vi "Decode.vi"(8 "Inputs":T1={"Frequency1"=2000.0, "Bit Duration in ms"=0.05, "Frequency2"=4000.0, "Amplitude Scale"=1.0, "Sampling Rate"=50000} {"Frequency2" format="%#_13g"; "Frequency1" format="%#_13g"}, 10 "Waveform Array":u16[](array[numeric])=array[20000 elements], 11 "Expected Characters":u16) -> (2 "string":string)   [LabVIEW 2021]
uses:
  <vilib>/Analysis/baseanly.llb/Mean (DBL).vi
  <vilib>/Analysis/NI_AALBase.lvlib
panel:
  out "size(s)":i32
  out "Array":bool[](array[boolean])
  out "Samples per bit":dbl
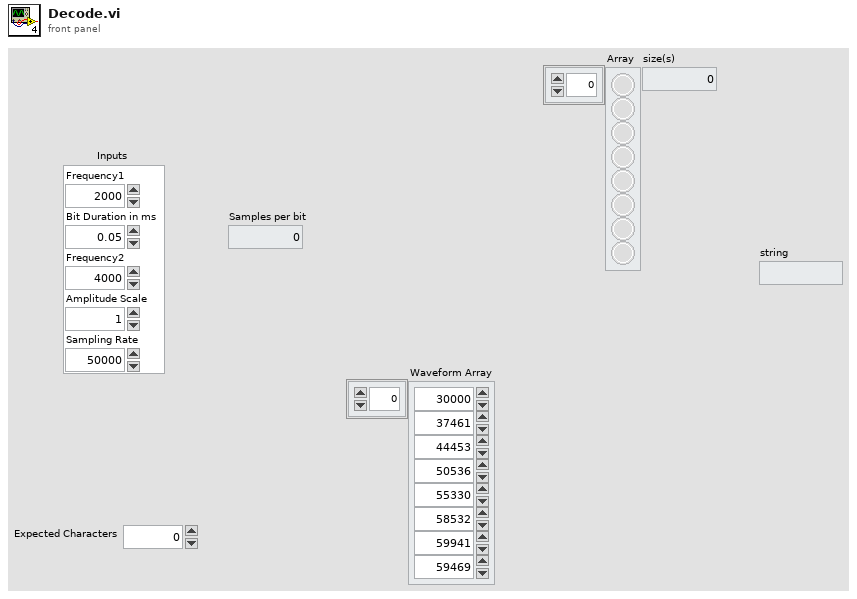
[diagram p1: front panel]
types:
  T1 = cluster{"Frequency1":dbl, "Bit Duration in ms":dbl, "Frequency2":dbl, "Amplitude Scale":dbl, "Sampling Rate":u32}
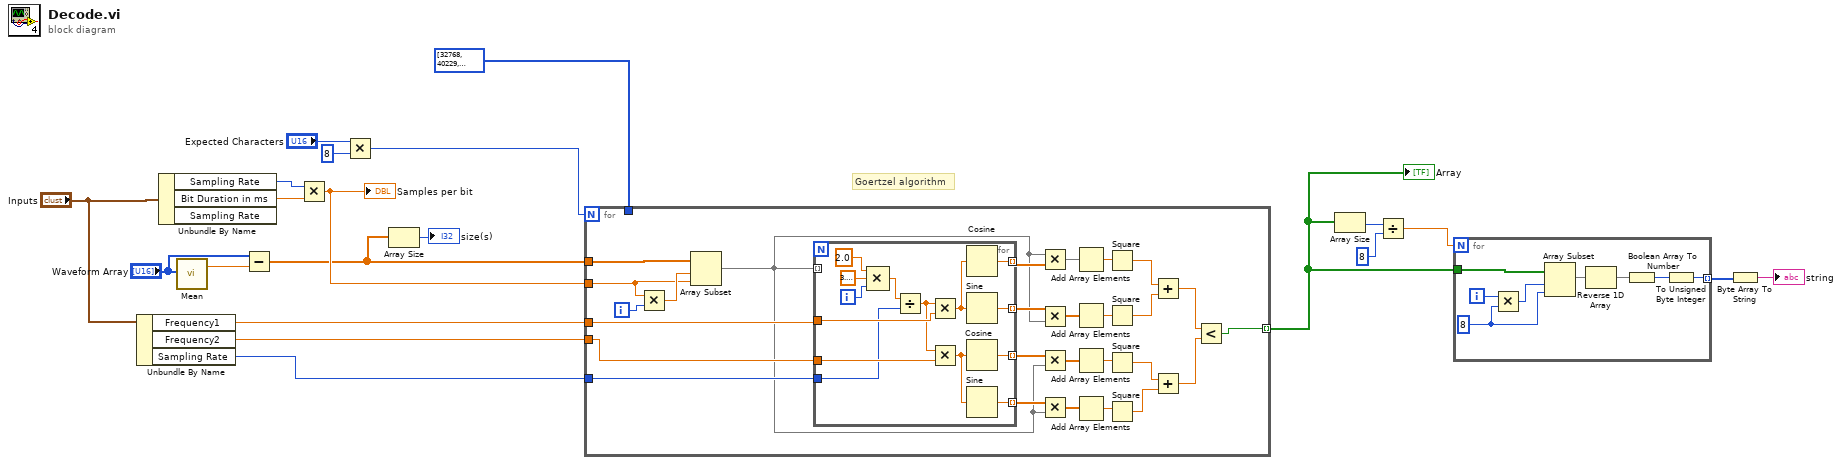
[diagram p0: block diagram]
diagram:
  # "Goertzel algorithm"
  n1 = Unbundle By Name("Inputs") -> ("Frequency1"=w15:dbl, "Frequency2"=w14:dbl, "Sampling Rate"=w13:u32)
  n2 = Unbundle By Name("Inputs") -> ("Sampling Rate"=w19:u32, "Bit Duration in ms"=w18:dbl)  [unwired: 1 out]
  n3 = call-poly <vilib>:"Mean.vi"("X"="Waveform Array") -> ("mean"=w20:dbl)  [unwired: 1 out]
  n4 = Subtract(x="Waveform Array", y=w20) -> (x-y=w6:dbl[])
  n5 = Multiply(x=w19, y=w18) -> (x*y=w17:dbl)
  "Samples per bit" <- w17
  n6 = Multiply(x="Expected Characters", y=u16 8) -> (x*y=w2:u16)
  n7 = Array Size(array=w6) -> (size(s)=→"size(s)":i32)
  n8 = for {
    N: w2 -> [_]
    tunnel: w6 -> [w48]
    tunnel: w17 -> [w45]
    tunnel: w15 -> [w43]
    tunnel: w14 -> [w44]
    tunnel: w13 -> [w42]
    tunnel: [w22] -> w12 mode=indexing
    tunnel: u16[] [32768, 40229, 47221, 53304, 58098, 61300, 62709, 62237, 59913, 55883, 50402, 43812, 36528, 29008, 21724, 15134, 9653, 5623, 3299, 2827, 4236, 7438, 12232, 18315, 25307, 32768, 40229, 47221, 53304, 58098, 61300, 62709, 62237, 59913, 55883, 50402, 43812, 36528, 29008, 21724, 15134, 9653, 5623, 3299, 2827, 4236, 7438, 12232, 18315, 25307, 32768, 40229, 47221, 53304, 58098, 61300, 62709, 62237, 59913, 55883, 50402, 43812, 36528, 29008, 21724, 15134, 9653, 5623, 3299, 2827, 4236, 7438, 12232, 18315, 25307, 32768, 40229, 47221, 53304, 58098, 61300, 62709, 62237, 59913, 55883, 50402, 43812, 36528, 29008, 21724, 15134, 9653, 5623, 3299, 2827, 4236, 7438, 12232, 18315, 25307, 32768, 40229, 47221, 53304, 58098, 61300, 62709, 62237, 59913, 55883, 50402, 43812, 36528, 29008, 21724, 15134, 9653, 5623, 3299, 2827, 4236, 7438, 12232, 18315, 25307, 32768, 40229, 47221, 53304, 58098, 61300, 62709, 62237, 59913, 55883, 50402, 43812, 36528, 29008, 21724, 15134, 9653, 5623, 3299, 2827, 4236, 7438, 12232, 18315, 25307, 32768, 40229, 47221, 53304, 58098, 61300, 62709, 62237, 59913, 55883, 50402, 43812, 36528, 29008, 21724, 15134, 9653, 5623, 3299, 2827, 4236, 7438, 12232, 18315, 25307, 32768, 40229, 47221, 53304, 58098, 61300, 62709, 62237, 59913, 55883, 50402, 43812, 36528, 29008, 21724, 15134, 9653, 5623, 3299, 2827, 4236, 7438, 12232, 18315, 25307, 32768, 40229, 47221, 53304, 58098, 61300, 62709, 62237, 59913, 55883, 50402, 43812, 36528, 29008, 21724, 15134, 9653, 5623, 3299, 2827, 4236, 7438, 12232, 18315, 25307, 32768, 40229, 47221, 53304, 58098, 61300, 62709, 62237, 59913, 55883, 50402, 43812, 36528, 29008, 21724, 15134, 9653, 5623, 3299, 2827, 4236, 7438, 12232, 18315, 25307, 32768, 40229, 47221, 53304, 58098, 61300, 62709, 62237, 59913, 55883, 50402, 43812, 36528, 29008, 21724, 15134, 9653, 5623, 3299, 2827, 4236, 7438, 12232, 18315, 25307, 32768, 40229, 47221, 53304, 58098, 61300, 62709, 62237, 59913, 55883, 50402, 43812, 36528, 29008, 21724, 15134, 9653, 5623, 3299, 2827, 4236, 7438, 12232, 18315, 25307, 32768, 40229, 47221, 53304, 58098, 61300, 62709, 62237, 59913, 55883, 50402, 43812, 36528, 29008, 21724, 15134, 9653, 5623, 3299, 2827, 4236, 7438, 12232, 18315, 25307, 32768, 40229, 47221, 53304, 58098, 61300, 62709, 62237, 59913, 55883, 50402, 43812, 36528, 29008, 21724, 15134, 9653, 5623, 3299, 2827, 4236, 7438, 12232, 18315, 25307, 32768, 40229, 47221, 53304, 58098, 61300, 62709, 62237, 59913, 55883, 50402, 43812, 36528, 29008, 21724, 15134, 9653, 5623, 3299, 2827, 4236, 7438, 12232, 18315, 25307, 32768, 40229, 47221, 53304, 58098, 61300, 62709, 62237, 59913, 55883, 50402, 43812, 36528, 29008, 21724, 15134, 9653, 5623, 3299, 2827, 4236, 7438, 12232, 18315, 25307, 32768, 40229, 47221, 53304, 58098, 61300, 62709, 62237, 59913, 55883, 50402, 43812, 36528, 29008, 21724, 15134, 9653, 5623, 3299, 2827, 4236, 7438, 12232, 18315, 25307, 32768, 40229, 47221, 53304, 58098, 61300, 62709, 62237, 59913, 55883, 50402, 43812, 36528, 29008, 21724, 15134, 9653, 5623, 3299, 2827, 4236, 7438, 12232, 18315, 25307, 32768, 40229, 47221, 53304, 58098, 61300, 62709, 62237, 59913, 55883, 50402, 43812, 36528, 29008, 21724, 15134, 9653, 5623, 3299, 2827, 4236, 7438, 12232, 18315, 25307, 32768, 40229, 47221, 53304, 58098, 61300, 62709, 62237, 59913, 55883, 50402, 43812, 36528, 29008, 21724, 15134, 9653, 5623, 3299, 2827, 4236, 7438, 12232, 18315, 25307, 32768, 40229, 47221, 53304, 58098, 61300, 62709, 62237, 59913, 55883, 50402, 43812, 36528, 29008, 21724, 15134, 9653, 5623, 3299, 2827, 4236, 7438, 12232, 18315, 25307, 32768, 40229, 47221, 53304, 58098, 61300, 62709, 62237, 59913, 55883, 50402, 43812, 36528, 29008, 21724, 15134, 9653, 5623, 3299, 2827, 4236, 7438, 12232, 18315, 25307, 32768, 40229, 47221, 53304, 58098, 61300, 62709, 62237, 59913, 55883, 50402, 43812, 36528, 29008, 21724, 15134, 9653, 5623, 3299, 2827, 4236, 7438, 12232, 18315, 25307, 32768, 40229, 47221, 53304, 58098, 61300, 62709, 62237, 59913, 55883, 50402, 43812, 36528, 29008, 21724, 15134, 9653, 5623, 3299, 2827, 4236, 7438, 12232, 18315, 25307, 32768, 40229, 47221, 53304, 58098, 61300, 62709, 62237, 59913, 55883, 50402, 43812, 36528, 29008, 21724, 15134, 9653, 5623, 3299, 2827, 4236, 7438, 12232, 18315, 25307, 32768, 40229, 47221, 53304, 58098, 61300, 62709, 62237, 59913, 55883, 50402, 43812, 36528, 29008, 21724, 15134, 9653, 5623, 3299, 2827, 4236, 7438, 12232, 18315, 25307, 32768, 40229, 47221, 53304, 58098, 61300, 62709, 62237, 59913, 55883, 50402, 43812, 36528, 29008, 21724, 15134, 9653, 5623, 3299, 2827, 4236, 7438, 12232, 18315, 25307, 32768, 40229, 47221, 53304, 58098, 61300, 62709, 62237, 59913, 55883, 50402, 43812, 36528, 29008, 21724, 15134, 9653, 5623, 3299, 2827, 4236, 7438, 12232, 18315, 25307, 32768, 40229, 47221, 53304, 58098, 61300, 62709, 62237, 59913, 55883, 50402, 43812, 36528, 29008, 21724, 15134, 9653, 5623, 3299, 2827, 4236, 7438, 12232, 18315, 25307, 32768, 40229, 47221, 53304, 58098, 61300, 62709, 62237, 59913, 55883, 50402, 43812, 36528, 29008, 21724, 15134, 9653, 5623, 3299, 2827, 4236, 7438, 12232, 18315, 25307, 32768, 40229, 47221, 53304, 58098, 61300, 62709, 62237, 59913, 55883, 50402, 43812, 36528, 29008, 21724, 15134, 9653, 5623, 3299, 2827, 4236, 7438, 12232, 18315, 25307, 32768, 40229, 47221, 53304, 58098, 61300, 62709, 62237, 59913, 55883, 50402, 43812, 36528, 29008, 21724, 15134, 9653, 5623, 3299, 2827, 4236, 7438, 12232, 18315, 25307, 32768, 40229, 47221, 53304, 58098, 61300, 62709, 62237, 59913, 55883, 50402, 43812, 36528, 29008, 21724, 15134, 9653, 5623, 3299, 2827, 4236, 7438, 12232, 18315, 25307, 32768, 40229, 47221, 53304, 58098, 61300, 62709, 62237, 59913, 55883, 50402, 43812, 36528, 29008, 21724, 15134, 9653, 5623, 3299, 2827, 4236, 7438, 12232, 18315, 25307, 32768, 40229, 47221, 53304, 58098, 61300, 62709, 62237, 59913, 55883, 50402, 43812, 36528, 29008, 21724, 15134, 9653, 5623, 3299, 2827, 4236, 7438, 12232, 18315, 25307, 32768, 40229, 47221, 53304, 58098, 61300, 62709, 62237, 59913, 55883, 50402, 43812, 36528, 29008, 21724, 15134, 9653, 5623, 3299, 2827, 4236, 7438, 12232, 18315, 25307, 32768, 40229, 47221, 53304, 58098, 61300, 62709, 62237, 59913, 55883, 50402, 43812, 36528, 29008, 21724, 15134, 9653, 5623, 3299, 2827, 4236, 7438, 12232, 18315, 25307, 32768, 40229, 47221, 53304, 58098, 61300, 62709, 62237, 59913, 55883, 50402, 43812, 36528, 29008, 21724, 15134, 9653, 5623, 3299, 2827, 4236, 7438, 12232, 18315, 25307, 32768, 40229, 47221, 53304, 58098, 61300, 62709, 62237, 59913, 55883, 50402, 43812, 36528, 29008, 21724, 15134, 9653, 5623, 3299, 2827, 4236, 7438, 12232, 18315, 25307, 32768, 40229, 47221, 53304, 58098, 61300, 62709, 62237, 59913, 55883, 50402, 43812, 36528, 29008, 21724, 15134, 9653, 5623, 3299, 2827, 4236, 7438, 12232, 18315, 25307, 32768, 40229, 47221, 53304, 58098, 61300, 62709, 62237, 59913, 55883, 50402, 43812, 36528, 29008, 21724, 15134, 9653, 5623, 3299, 2827, 4236, 7438, 12232, 18315, 25307, 32768, 40229, 47221, 53304, 58098, 61300, 62709, 62237, 59913, 55883, 50402, 43812, 36528, 29008, 21724, 15134, 9653, 5623, 3299, 2827, 4236, 7438, 12232, 18315, 25307, 32768, 40229, 47221, 53304, 58098, 61300, 62709, 62237, 59913, 55883, 50402, 43812, 36528, 29008, 21724, 15134, 9653, 5623, 3299, 2827, 4236, 7438, 12232, 18315, 25307, 32768, 40229, 47221, 53304, 58098, 61300, 62709, 62237, 59913, 55883, 50402, 43812, 36528, 29008, 21724, 15134, 9653, 5623, 3299, 2827, 4236, 7438, 12232, 18315, 25307, 32768, 40229, 47221, 53304, 58098, 61300, 62709, 62237, 59913, 55883, 50402, 43812, 36528, 29008, 21724, 15134, 9653, 5623, 3299, 2827, 4236, 7438, 12232, 18315, 25307, 32768, 40229, 47221, 53304, 58098, 61300, 62709, 62237, 59913, 55883, 50402, 43812, 36528, 29008, 21724, 15134, 9653, 5623, 3299, 2827, 4236, 7438, 12232, 18315, 25307, 32768, 40229, 47221, 53304, 58098, 61300, 62709, 62237, 59913, 55883, 50402, 43812, 36528, 29008, 21724, 15134, 9653, 5623, 3299, 2827, 4236, 7438, 12232, 18315, 25307, 32768, 40229, 47221, 53304, 58098, 61300, 62709, 62237, 59913, 55883, 50402, 43812, 36528, 29008, 21724, 15134, 9653, 5623, 3299, 2827, 4236, 7438, 12232, 18315, 25307, 32768, 40229, 47221, 53304, 58098, 61300, 62709, 62237, 59913, 55883, 50402, 43812, 36528, 29008, 21724, 15134, 9653, 5623, 3299, 2827, 4236, 7438, 12232, 18315, 25307, 32768, 40229, 47221, 53304, 58098, 61300, 62709, 62237, 59913, 55883, 50402, 43812, 36528, 29008, 21724, 15134, 9653, 5623, 3299, 2827, 4236, 7438, 12232, 18315, 25307, 32768, 40229, 47221, 53304, 58098, 61300, 62709, 62237, 59913, 55883, 50402, 43812, 36528, 29008, 21724, 15134, 9653, 5623, 3299, 2827, 4236, 7438, 12232, 18315, 25307, 32768, 40229, 47221, 53304, 58098, 61300, 62709, 62237, 59913, 55883, 50402, 43812, 36528, 29008, 21724, 15134, 9653, 5623, 3299, 2827, 4236, 7438, 12232, 18315, 25307, 32768, 40229, 47221, 53304, 58098, 61300, 62709, 62237, 59913, 55883, 50402, 43812, 36528, 29008, 21724, 15134, 9653, 5623, 3299, 2827, 4236, 7438, 12232, 18315, 25307, 32768, 40229, 47221, 53304, 58098, 61300, 62709, 62237, 59913, 55883, 50402, 43812, 36528, 29008, 21724, 15134, 9653, 5623, 3299, 2827, 4236, 7438, 12232, 18315, 25307, 32768, 40229, 47221, 53304, 58098, 61300, 62709, 62237, 59913, 55883, 50402, 43812, 36528, 29008, 21724, 15134, 9653, 5623, 3299, 2827, 4236, 7438, 12232, 18315, 25307, 32768, 40229, 47221, 53304, 58098, 61300, 62709, 62237, 59913, 55883, 50402, 43812, 36528, 29008, 21724, 15134, 9653, 5623, 3299, 2827, 4236, 7438, 12232, 18315, 25307, 32768, 40229, 47221, 53304, 58098, 61300, 62709, 62237, 59913, 55883, 50402, 43812, 36528, 29008, 21724, 15134, 9653, 5623, 3299, 2827, 4236, 7438, 12232, 18315, 25307, 32768, 40229, 47221, 53304, 58098, 61300, 62709, 62237, 59913, 55883, 50402, 43812, 36528, 29008, 21724, 15134, 9653, 5623, 3299, 2827, 4236, 7438, 12232, 18315, 25307, 32768, 40229, 47221, 53304, 58098, 61300, 62709, 62237, 59913, 55883, 50402, 43812, 36528, 29008, 21724, 15134, 9653, 5623, 3299, 2827, 4236, 7438, 12232, 18315, 25307, 32768, 40229, 47221, 53304, 58098, 61300, 62709, 62237, 59913, 55883, 50402, 43812, 36528, 29008, 21724, 15134, 9653, 5623, 3299, 2827, 4236, 7438, 12232, 18315, 25307, 32768, 40229, 47221, 53304, 58098, 61300, 62709, 62237, 59913, 55883, 50402, 43812, 36528, 29008, 21724, 15134, 9653, 5623, 3299, 2827, 4236, 7438, 12232, 18315, 25307, 32768, 40229, 47221, 53304, 58098, 61300, 62709, 62237, 59913, 55883, 50402, 43812, 36528, 29008, 21724, 15134, 9653, 5623, 3299, 2827, 4236, 7438, 12232, 18315, 25307, 32768, 40229, 47221, 53304, 58098, 61300, 62709, 62237, 59913, 55883, 50402, 43812, 36528, 29008, 21724, 15134, 9653, 5623, 3299, 2827, 4236, 7438, 12232, 18315, 25307, 32768, 40229, 47221, 53304, 58098, 61300, 62709, 62237, 59913, 55883, 50402, 43812, 36528, 29008, 21724, 15134, 9653, 5623, 3299, 2827, 4236, 7438, 12232, 18315, 25307, 32768, 40229, 47221, 53304, 58098, 61300, 62709, 62237, 59913, 55883, 50402, 43812, 36528, 29008, 21724, 15134, 9653, 5623, 3299, 2827, 4236, 7438, 12232, 18315, 25307, 32768, 40229, 47221, 53304, 58098, 61300, 62709, 62237, 59913, 55883, 50402, 43812, 36528, 29008, 21724, 15134, 9653, 5623, 3299, 2827, 4236, 7438, 12232, 18315, 25307, 32768, 40229, 47221, 53304, 58098, 61300, 62709, 62237, 59913, 55883, 50402, 43812, 36528, 29008, 21724, 15134, 9653, 5623, 3299, 2827, 4236, 7438, 12232, 18315, 25307, 32768, 40229, 47221, 53304, 58098, 61300, 62709, 62237, 59913, 55883, 50402, 43812, 36528, 29008, 21724, 15134, 9653, 5623, 3299, 2827, 4236, 7438, 12232, 18315, 25307, 32768, 40229, 47221, 53304, 58098, 61300, 62709, 62237, 59913, 55883, 50402, 43812, 36528, 29008, 21724, 15134, 9653, 5623, 3299, 2827, 4236, 7438, 12232, 18315, 25307, 32768, 40229, 47221, 53304, 58098, 61300, 62709, 62237, 59913, 55883, 50402, 43812, 36528, 29008, 21724, 15134, 9653, 5623, 3299, 2827, 4236, 7438, 12232, 18315, 25307, 32768, 40229, 47221, 53304, 58098, 61300, 62709, 62237, 59913, 55883, 50402, 43812, 36528, 29008, 21724, 15134, 9653, 5623, 3299, 2827, 4236, 7438, 12232, 18315, 25307, 32768, 40229, 47221, 53304, 58098, 61300, 62709, 62237, 59913, 55883, 50402, 43812, 36528, 29008, 21724, 15134, 9653, 5623, 3299, 2827, 4236, 7438, 12232, 18315, 25307, 32768, 40229, 47221, 53304, 58098, 61300, 62709, 62237, 59913, 55883, 50402, 43812, 36528, 29008, 21724, 15134, 9653, 5623, 3299, 2827, 4236, 7438, 12232, 18315, 25307, 32768, 40229, 47221, 53304, 58098, 61300, 62709, 62237, 59913, 55883, 50402, 43812, 36528, 29008, 21724, 15134, 9653, 5623, 3299, 2827, 4236, 7438, 12232, 18315, 25307, 32768, 40229, 47221, 53304, 58098, 61300, 62709, 62237, 59913, 55883, 50402, 43812, 36528, 29008, 21724, 15134, 9653, 5623, 3299, 2827, 4236, 7438, 12232, 18315, 25307, 32768, 40229, 47221, 53304, 58098, 61300, 62709, 62237, 59913, 55883, 50402, 43812, 36528, 29008, 21724, 15134, 9653, 5623, 3299, 2827, 4236, 7438, 12232, 18315, 25307, 32768, 40229, 47221, 53304, 58098, 61300, 62709, 62237, 59913, 55883, 50402, 43812, 36528, 29008, 21724, 15134, 9653, 5623, 3299, 2827, 4236, 7438, 12232, 18315, 25307, 32768, 40229, 47221, 53304, 58098, 61300, 62709, 62237, 59913, 55883, 50402, 43812, 36528, 29008, 21724, 15134, 9653, 5623, 3299, 2827, 4236, 7438, 12232, 18315, 25307, 32768, 40229, 47221, 53304, 58098, 61300, 62709, 62237, 59913, 55883, 50402, 43812, 36528, 29008, 21724, 15134, 9653, 5623, 3299, 2827, 4236, 7438, 12232, 18315, 25307, 32768, 40229, 47221, 53304, 58098, 61300, 62709, 62237, 59913, 55883, 50402, 43812, 36528, 29008, 21724, 15134, 9653, 5623, 3299, 2827, 4236, 7438, 12232, 18315, 25307, 32768, 40229, 47221, 53304, 58098, 61300, 62709, 62237, 59913, 55883, 50402, 43812, 36528, 29008, 21724, 15134, 9653, 5623, 3299, 2827, 4236, 7438, 12232, 18315, 25307, 32768, 40229, 47221, 53304, 58098, 61300, 62709, 62237, 59913, 55883, 50402, 43812, 36528, 29008, 21724, 15134, 9653, 5623, 3299, 2827, 4236, 7438, 12232] ("Waveform Array") -> [_]
    i -> [w47]
    n9 = Multiply(x=w45, y=w47) -> (x*y=w46:dbl)
    n10 = Array Subset(array=w48, index=w46, length=w45) -> (w37:dbl[])
    n11 = for {
      tunnel: w37 -> [_] mode=indexing
      tunnel: w43 -> [w59]
      tunnel: w44 -> [w58]
      tunnel: [w53] -> w41 mode=indexing
      tunnel: [w52] -> w40 mode=indexing
      tunnel: [w51] -> w39 mode=indexing
      tunnel: [w50] -> w38 mode=indexing
      tunnel: w42 -> [w49]
      i -> [w60]
      n12 = Compound Arithmetic op=MULTIPLY(2.0 ("x"), 3.141592653589793, w60) -> (w57:dbl)
      n13 = Divide(x=w57, y=w49) -> (x/y=w54:dbl)
      n14 = Multiply(x=w54, y=w59) -> (x*y=w56:dbl)
      n15 = Multiply(x=w54, y=w58) -> (x*y=w55:dbl)
      n16 = Cosine(x=w56) -> (cos(x)=w53:dbl)
      n17 = Sine(x=w56) -> (sin(x)=w52:dbl)
      n18 = Cosine(x=w55) -> (cos(x)=w51:dbl)
      n19 = Sine(x=w55) -> (sin(x)=w50:dbl)
    }
    n20 = Multiply(x=w37, y=w41) -> (x*y=w36:dbl[])
    n21 = Multiply(x=w40, y=w37) -> (x*y=w35:dbl[])
    n22 = Multiply(x=w39, y=w37) -> (x*y=w34:dbl[])
    n23 = Multiply(x=w38, y=w37) -> (x*y=w33:dbl[])
    n24 = Add Array Elements(numeric array=w36) -> (sum=w32:dbl)
    n25 = Add Array Elements(numeric array=w35) -> (sum=w31:dbl)
    n26 = Add Array Elements(numeric array=w34) -> (sum=w30:dbl)
    n27 = Add Array Elements(numeric array=w33) -> (sum=w29:dbl)
    n28 = Square(x=w32) -> (x^2=w27:dbl)
    n29 = Square(x=w31) -> (x^2=w28:dbl)
    n30 = Square(x=w30) -> (x^2=w26:dbl)
    n31 = Square(x=w29) -> (x^2=w25:dbl)
    n32 = Add(x=w27, y=w28) -> (x+y=w24:dbl)
    n33 = Add(x=w26, y=w25) -> (x+y=w23:dbl)
    n34 = Less?(x=w24, y=w23) -> (x < y?=w22:bool)
  }
  "Array" <- w12
  n35 = Array Size(array=w12) -> (size(s)=w11:i32)
  n36 = Divide(x=w11, y=8) -> (x/y=w9:dbl)
  n37 = for {
    N: w9 -> [_]
    tunnel: w12 -> [w70]
    tunnel: [w64] -> w8 mode=indexing
    i -> [w69]
    w67 = u8 8 ("y")
    n38 = Multiply(x=w69, y=w67) -> (x*y=w68:i32)
    n39 = Array Subset(array=w70, index=w68, length=w67) -> (w66:bool[])
    n40 = Reverse 1D Array(array=w66) -> (reversed array=w63:bool[])
    n41 = Boolean Array To Number(Boolean array=w63) -> (number=w65:u32)
    n42 = To Unsigned Byte Integer(number=w65) -> (unsigned 8bit integer=w64:u8)
  }
  n43 = Byte Array To String(unsigned byte array=w8) -> (string=→"string":string)
